vi "Park_from_park.vi"(1 "offset Y":dbl, 3 "offset X":dbl, 4 "Line_start":i32, 5 "Range":dbl=10.0, 6 "Pixels":i32=256, 7 "dwell":dbl=1.0) -> (0 "X and Y":waveform(dbl)[](array[waveform]))   [LabVIEW 2016]
panel:
  out "Waveform Graph":waveform(dbl)[](graph)
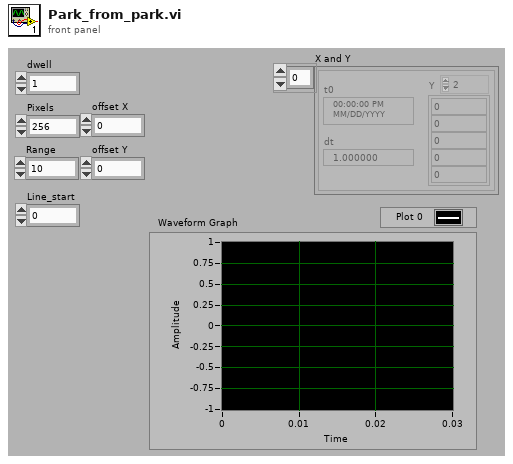
[diagram p1: front panel]
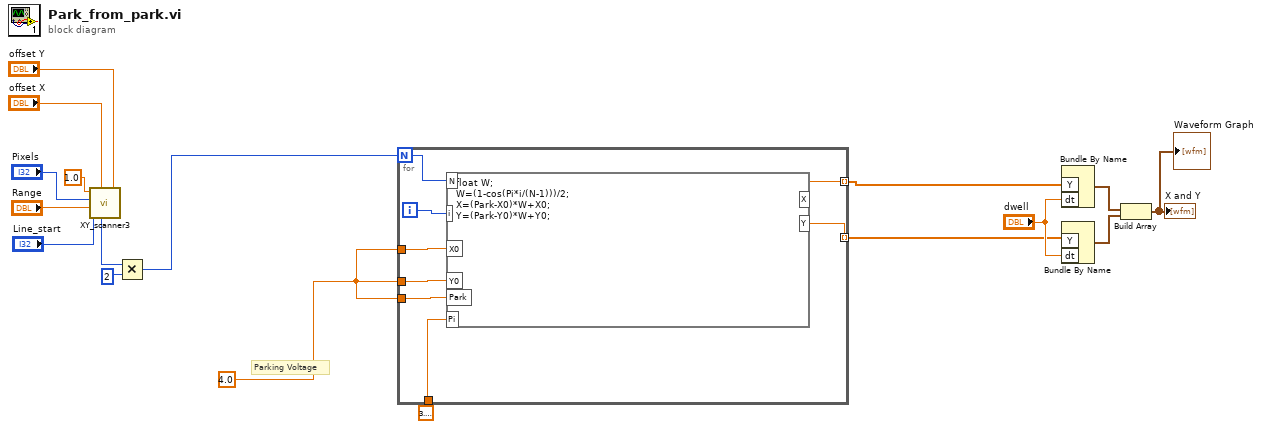
[diagram p0: block diagram]
diagram:
  w1 = 4.0 ("input variable")
  # "Parking Voltage"
  n1 = call "XY_scanner3.vi"("offset Y"="offset Y", "offset X"="offset X", "Line_start"="Line_start", "Range"="Range", "Pixels"="Pixels", "dwell"=1.0) -> ("scanPix"=w9:i32)  [unwired: 3 out]
  n2 = Multiply(x=w9, y=2) -> (x*y=w8:i32)
  n3 = for {
    N: w8 -> [w24]
    tunnel: 3.141592653589793 -> [w23]
    tunnel: [w22] -> w2 mode=indexing
    tunnel: [w21] -> w3 mode=indexing
    tunnel: w1 -> [w20]
    tunnel: w1 -> [w19]
    tunnel: w1 -> [w18]
    i -> [w25]
    n4 = formula code="float W;\nW=(1-cos(Pi*i/(N-1)))/2;\nX=(Park-X0)*W+X0;\nY=(Park-Y0)*W+Y0;"("N"=w24, "i"=w25, "Pi"=w23, "X0"=w20, "Y0"=w19, "Park"=w18) -> ("X"=w22:dbl, "Y"=w21:dbl)
  }
  n5 = Bundle By Name("Y"=w2, "dt"="dwell") -> (w14:waveform(dbl))  [unwired: 1 in]
  n6 = Bundle By Name("Y"=w3, "dt"="dwell") -> (w13:waveform(dbl))  [unwired: 1 in]
  n7 = Build Array(w14, w13) -> (→"X and Y" →"Waveform Graph":waveform(dbl)[])
